vi "Get Device Information.vi"(8 "error in":errorcluster, 10 "RIO Target in":refnum<class "RIO Target.lvclass">, 11 "Bus in":refnum<class "Bus.lvclass">) -> (0 "error out":errorcluster, 1 "Enable Lines":string[](array[string]), 2 "Chip Select Lines":string[](array[string]), 3 "Bus out":refnum<class "Bus.lvclass">, 5 "Device Information Array":T1[](array[typedef]))   [LabVIEW 2014, in "Bus.lvclass"]
uses:
  Bus.lvclass
  Scripting/Initialization Scripting/State Machine/Controls/Device Information.ctl
  <vilib>/LabVIEW Icon API/API_Text.ctl
  RIO Target/RIO Target.lvclass
  <vilib>/NI/Configuration Framework/Node/NISE_CEF_Node.lvclass/NISE_CEF_Node.ctl
  Device node/Device.lvclass
  Device Configuration/Device Configuration.lvclass
  Device Configuration/Device Configuration.lvclass/Device Configuration.ctl
  <vilib>/NI/Configuration Framework/serializable configuration/read metadata property.vi
  <vilib>/NI/Configuration Framework/Node/NISE_CEF_Node.lvclass
  <vilib>/NI/Configuration Framework/serializable configuration/NISE_CEF_serializable configuration.lvclass
  <vilib>/LabVIEW Icon API/LabVIEW Icon API.lvlib
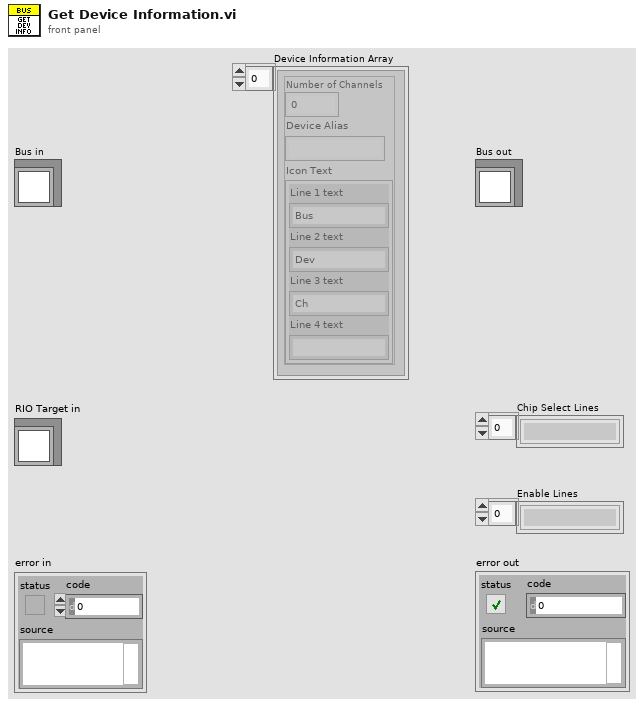
[diagram p1: front panel]
types:
  T1 = typedef "Device Information.ctl" = cluster{"Number of Channels":i32, "Device Alias":string, "Icon Text":T2}
  T2 = typedef "LabVIEW Icon API.lvlib/API_Text.ctl" = cluster{"Line 1 text":string, "Line 2 text":string, "Line 3 text":string, "Line 4 text":string}
  T3 = typedef "NISE_CEF_Node.lvclass/NodeRef.ctl" = refnum<data-value>
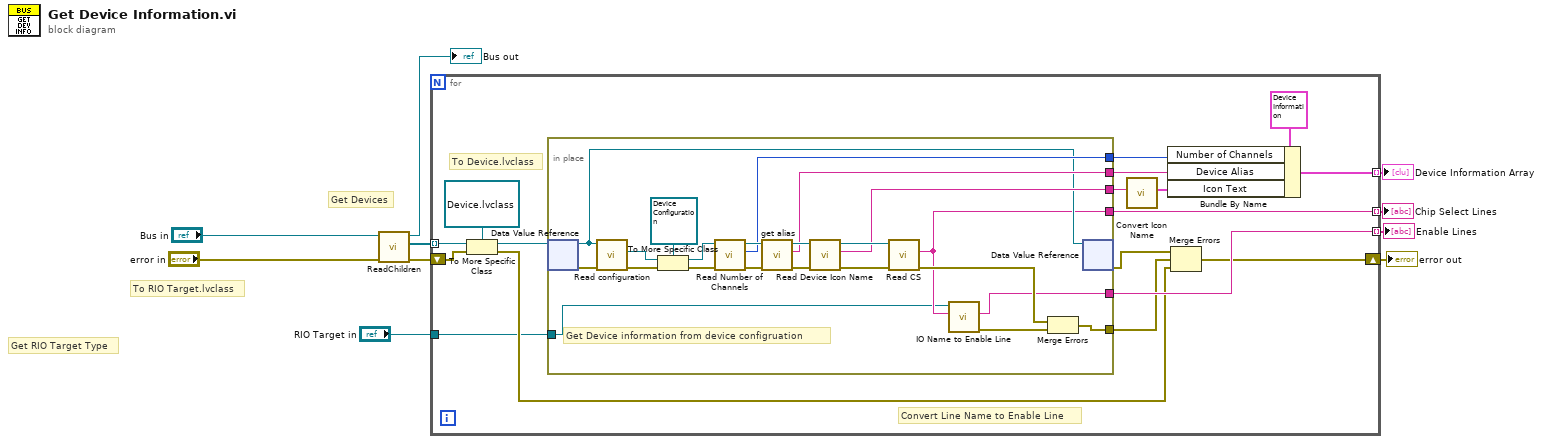
[diagram p0: block diagram]
diagram:
  # "Get RIO Target Type"
  # "To RIO Target.lvclass"
  # "Get Devices"
  n1 = call <vilib>:"ReadChildren.vi"("error in"="error in", "node in"="Bus in") -> ("error out"=w10:errorcluster, "output array"=w8:T3[], "node out"=→"Bus out":refnum<class "Bus.lvclass">)  [unwired: 7 in]
  n2 = for {
    tunnel: w8 -> [w27] mode=indexing
    tunnel: [w23] -> w9 mode=indexing
    shift-right: [w17] -> w5
    shift-left: w10 -> [w22]
    tunnel: [w19] -> w6 mode=indexing
    tunnel: [w14] -> w4 mode=indexing
    tunnel: "RIO Target in" -> [w13]
    # "Convert Line Name to Enable Line"
    # "To Device.lvclass"
    n3 = To More Specific Class(target class=refnum<data-value> refnum ("data value reference"), reference=w27, error in=w22) -> (specific class reference=w25:refnum<data-value>, error out=w15:errorcluster)
    n4 = in-place {
      in-place-border: [w35] -> w19
      in-place-border: [w34] -> w16
      in-place-border: [w33] -> w21
      in-place-border: [w32] -> w20
      in-place-border: [w31] -> w12
      in-place-border: [w29] -> w14
      in-place-border: w13 -> [w28]
      # "Get Device information from device configruation"
      n5 = in-place-dvr #1(w25) -> (w30:refnum<class "Device.lvclass">, w46:errorcluster)
      n6 = call-dynamic "Read configuration.vi"("error in"=w46, "Device in"=w30) -> ("error out"=w45:errorcluster, "configuration"=w49:refnum<class "NISE_CEF_serializable configuration.lvclass">)  [unwired: 7 in, 1 out]
      n7 = To More Specific Class(target class=refnum<class "Device Configuration.lvclass"> refnum ("Device Configuration.lvclass"), reference=w49, error in=w45) -> (specific class reference=w47:refnum<class "Device Configuration.lvclass">, error out=w44:errorcluster)
      n8 = call "Read Number of Channels.vi"("error in (no error)"=w44, "Device Configuration in"=w47) -> ("error out"=w40:errorcluster, "Number of Channels"=w33:u32, "Device Configuration out"=w41:refnum<class "Device Configuration.lvclass">)  [unwired: 7 in]
      n9 = call <vilib>:"get alias.vi"("error in"=w40, "configuration in"=w41) -> ("error out"=w42:errorcluster, "alias"=w32:string, "configuration out"=w43:refnum<class "Device Configuration.lvclass">)  [unwired: 7 in]
      n10 = call "Read Device Icon Name.vi"("error in (no error)"=w42, "Device Configuration in"=w43) -> ("error out"=w38:errorcluster, "Device Icon Name"=w31:string, "Device Configuration out"=w39:refnum<class "Device Configuration.lvclass">)  [unwired: 7 in]
      n11 = call "Read CS.vi"("error in (no error)"=w38, "Device Configuration in"=w39) -> ("error out"=w37:errorcluster, "CS"=w29:string)  [unwired: 7 in, 1 out]
      n12 = call-dynamic "IO Name to Enable Line.vi"("IO Name"=w29, "RIO Target in"=w28) -> ("error out"=w36:errorcluster, "Enable Line"=w35:string)  [unwired: 7 in, 1 out]
      n13 = Merge Errors(w37, w36) -> (w34:errorcluster)
      n14 = in-place-dvr #1(w30) -> (w18:errorcluster)  [unwired: 1 out]
    }
    n15 = call "Convert Icon Name.vi"("Device Icon Name"=w12) -> ("Icon Text"=w11:T2)  [unwired: 10 in]
    n16 = Bundle By Name(cluster=T1 {"Number of Channels"=1, "Device Alias"="", "Icon Text"={"Line 1 text"="Bus", "Line 2 text"="Dev", "Line 3 text"="Ch", "Line 4 text"=""}} ("Device Information"), "Number of Channels"=w21, "Device Alias"=w20, "Icon Text"=w11) -> (w23:T1)
    n17 = Merge Errors(w18, w16, w15) -> (w17:errorcluster)
  }
  "Device Information Array" <- w9
  "Enable Lines" <- w6
  "error out" <- w5
  "Chip Select Lines" <- w4
